vi "Acquire SFTP Handle.vi"(8 "error in (no error)":errorcluster, 11 "sftp handle":T1) -> (0 "error out":errorcluster, 2 "LIBSSH2_SFTP_HANDLE*":u64)   [LabVIEW 2013, in "libssh2.lvlib"]
uses:
  libssh2.lvlib
  SFTP Handle Refnum.ctl
  Acquire Session.vi
  Read SFTP Refnum.vi
  <vilib>/Utility/semaphor.llb/Acquire Semaphore.vi
  Read Session Refnum.vi
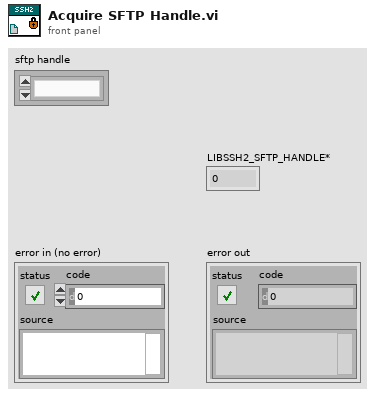
[diagram p1: front panel]
types:
  T1 = typedef "libssh2.lvlib/SFTP Handle Refnum.ctl" = refnum<k1>
  T2 = typedef "libssh2.lvlib/SFTP Refnum.ctl" = refnum<k1>
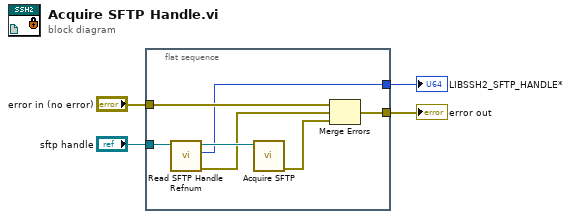
[diagram p0: block diagram]
diagram:
  n1 = flat-sequence {
    tunnel: [w8] -> w4
    tunnel: "error in (no error)" -> [w7]
    tunnel: "sftp handle" -> [w6]
    tunnel: [w5] -> w1
    frame #0 {
      n2 = call "Read SFTP Handle Refnum.vi"("sftp handle"=w6) -> ("error out"=w10:errorcluster, "LIBSSH2_SFTP_HANDLE*"=w5:u64, "sftp"=w11:T2)  [unwired: 8 in]
      n3 = call "Acquire SFTP.vi"("sftp"=w11) -> ("error out"=w9:errorcluster)  [unwired: 9 in, 1 out]
      n4 = Merge Errors(w7, w10, w9) -> (w8:errorcluster)
    }
  }
  "error out" <- w4
  "LIBSSH2_SFTP_HANDLE*" <- w1
